vi "DSF.Shared.Configuration.Get Custom Parameters.vi"(11 "Configuration in":refnum<class "DSF.Shared.Configuration.lvclass">) -> (2 "custom parameters":variant, 3 "Configuration out":refnum<class "DSF.Shared.Configuration.lvclass">)   [LabVIEW 2017, in "DSF.Engine.lvlib" / "DSF.Shared.Configuration.lvclass"]
uses:
  DSF.Shared.Configuration.lvclass
  DSF.Shared.Configuration.lvclass/DSF.Shared.Configuration.ctl
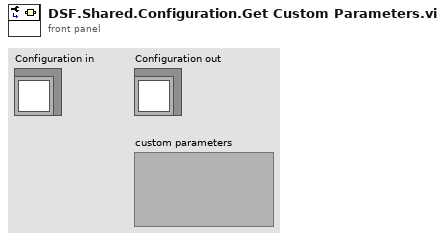
[diagram p1: front panel]
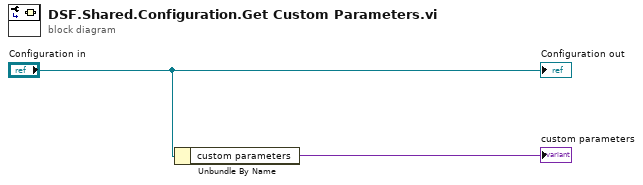
[diagram p0: block diagram]
diagram:
  n1 = Unbundle By Name("Configuration in") -> ("custom parameters"=→"custom parameters":variant)
  "Configuration out" <- "Configuration in"
